vi "Initialise.vi"(8 "error in (no error)":errorcluster, 10 "Message in":refnum<class "InitialiseMessage.lvclass">, 11 "BMC in":refnum<class "BMC.lvclass">) -> (0 "error out":errorcluster, 3 "BMC out":refnum<class "BMC.lvclass">)   [LabVIEW 2012, in "BMC.lvclass"]
doc: "This method is called when an initialise message is received. It mainly initialises the RabbitMQ connectivity. \n\nOverride this method when your component needs special initialisation (e.g. of software or hardware resources). In that case, don't forget to call the parent for proper implementation. If your component owns subcomponents, they count as resources, so you have to initialise them by calling their own initialise functions"
uses:
  BMC.lvclass
  Murmex/LabVIEW/Murmex/Murmex/Murmex.lvclass
  Murmex/LabVIEW/Murmex/InitialiseMessage/InitialiseMessage.lvclass
panel:
  # "This method is called when the INTIALISE\ntrigger is sent. \n\nOverride this method when your component needs to\nrespond to this trigger. \n\nCall parent for proper implementation"
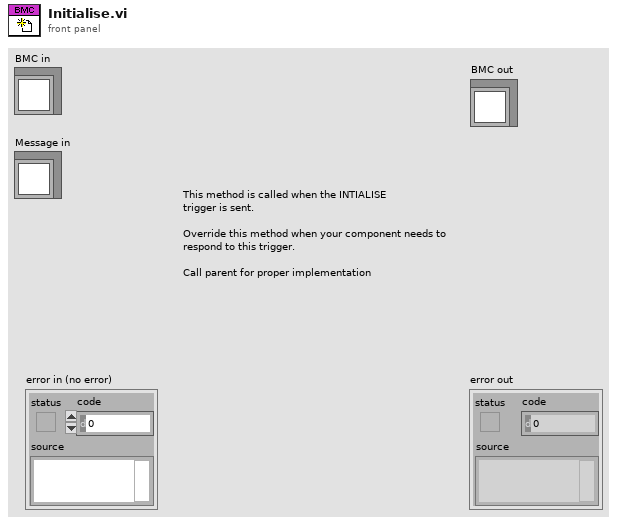
[diagram p1: front panel]
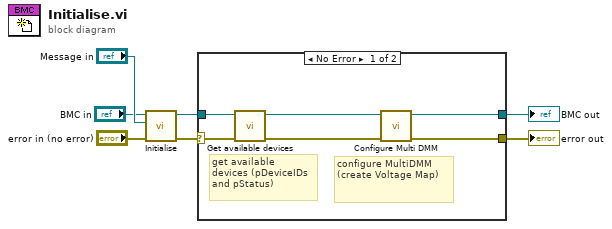
[diagram p0: block diagram]
diagram:
  n1 = call-parent "Initialise.vi"("error in (no error)"="error in (no error)", "Message in"="Message in", "Murmex in"="BMC in") -> ("error out"=w4:errorcluster, "Murmex out"=w2:refnum<class "BMC.lvclass">)  [unwired: 7 in]
  n2 = case shown="No Error" w4 {
    selector: w4 -> [w9 w15]
    tunnel: [w12 w15] -> w3
    tunnel: w2 -> [w8 w14]
    tunnel: [w10 w14] -> w1
    frame No Error {
      # "configure MultiDMM \n(create Voltage Map)"
      # "get available\ndevices (pDeviceIDs\nand pStatus)"
      n3 = call-dynamic "Get available devices.vi"("error in (no error)"=w9, "BMC in"=w8) -> ("error out"=w13:errorcluster, "BMC out"=w11:refnum<class "BMC.lvclass">)  [unwired: 8 in]
      n4 = call-dynamic "Configure Multi DMM.vi"("error in (no error)"=w13, "BMC in"=w11) -> ("error out"=w12:errorcluster, "BMC out"=w10:refnum<class "BMC.lvclass">)  [unwired: 8 in]
    }
    frame Error {
    }
  }
  "error out" <- w3
  "BMC out" <- w1
